vi "Construct.vi"(0 "iUser Configuration Manager in":refnum<class "iUser Configuration Manager.lvclass">, 5 "Encryption Type":refnum<class "iEncryption.lvclass">, 11 "error in (no error)":errorcluster) -> (4 "iUser Configuration Manager out":refnum<class "iUser Configuration Manager.lvclass">, 15 "error out":errorcluster)   [LabVIEW 2019, in "User Configuration Manager.lvlib" / "iUser Configuration Manager.lvclass"]
uses:
  <vilib>/gpm_packages/@cs/user-manager/Source/iUser Configuration Manager/iUser Configuration Manager.lvclass
  <vilib>/gpm_packages/@cs/user-manager/Source/iEncryption/iEncryption.lvclass
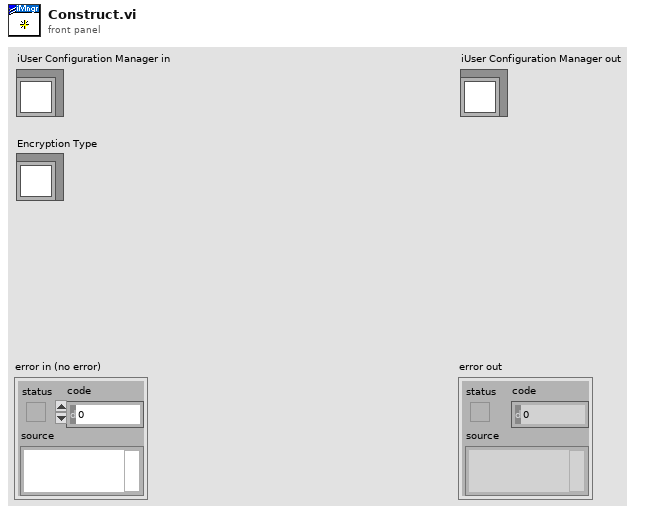
[diagram p1: front panel]
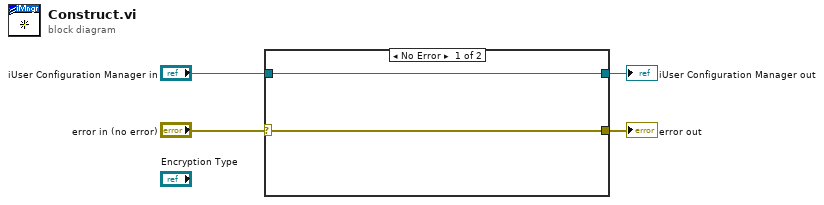
[diagram p0: block diagram]
diagram:
  n1 = case shown="No Error" "error in (no error)" {
    selector: "error in (no error)" -> [w5 w8]
    tunnel: [w5 w8] -> w3
    tunnel: [w6 w7] -> w1
    tunnel: "iUser Configuration Manager in" -> [w6 w7]
    frame No Error {
    }
    frame Error {
    }
  }
  "error out" <- w3
  "iUser Configuration Manager out" <- w1
